vi "SelectDailyData.vi"(8 "Shift":string="中", 10 "Begin_date":string, 11 "End_date":string) -> (2 "output array":string[][](array[string]))   [LabVIEW 2012]
uses:
  <vilib>/addons/database/Auxilliary.llb/DB Tools Cursor Type.ctl
  Global1.vi
  <vilib>/addons/database/Connection.llb/DB Tools Open Connec (Path).vi
  <vilib>/addons/database/Connection.llb/Conn Execute.vi
  <vilib>/addons/database/Recordset.llb/Rec Fetch Recordset Data (R).vi
  <vilib>/addons/database/Recordset.llb/Rec Destroy - Connection.vi
  <vilib>/addons/database/_DB Variant To Data/Database Variant To Data.xnode
  <vilib>/addons/database/NI_Database_API.lvlib
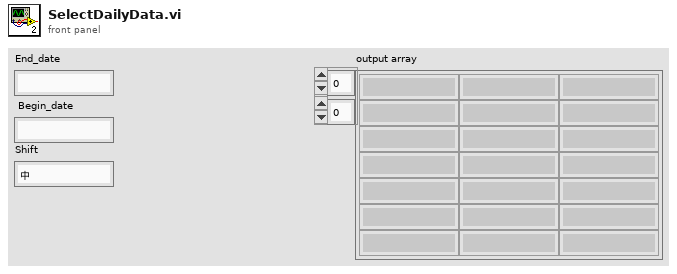
[diagram p1: front panel]
types:
  T1 = typedef "NI_Database_API.lvlib/DB Tools Cursor Type.ctl" = enum16{"forward-only", "keyset", "dynamic", "static"}
  T2 = typedef "NI_Database_API.lvlib/Conn ObjectReference.ctl" = refnum<k1>
  T3 = typedef "NI_Database_API.lvlib/Rec ObjectReference.ctl" = refnum<k1>
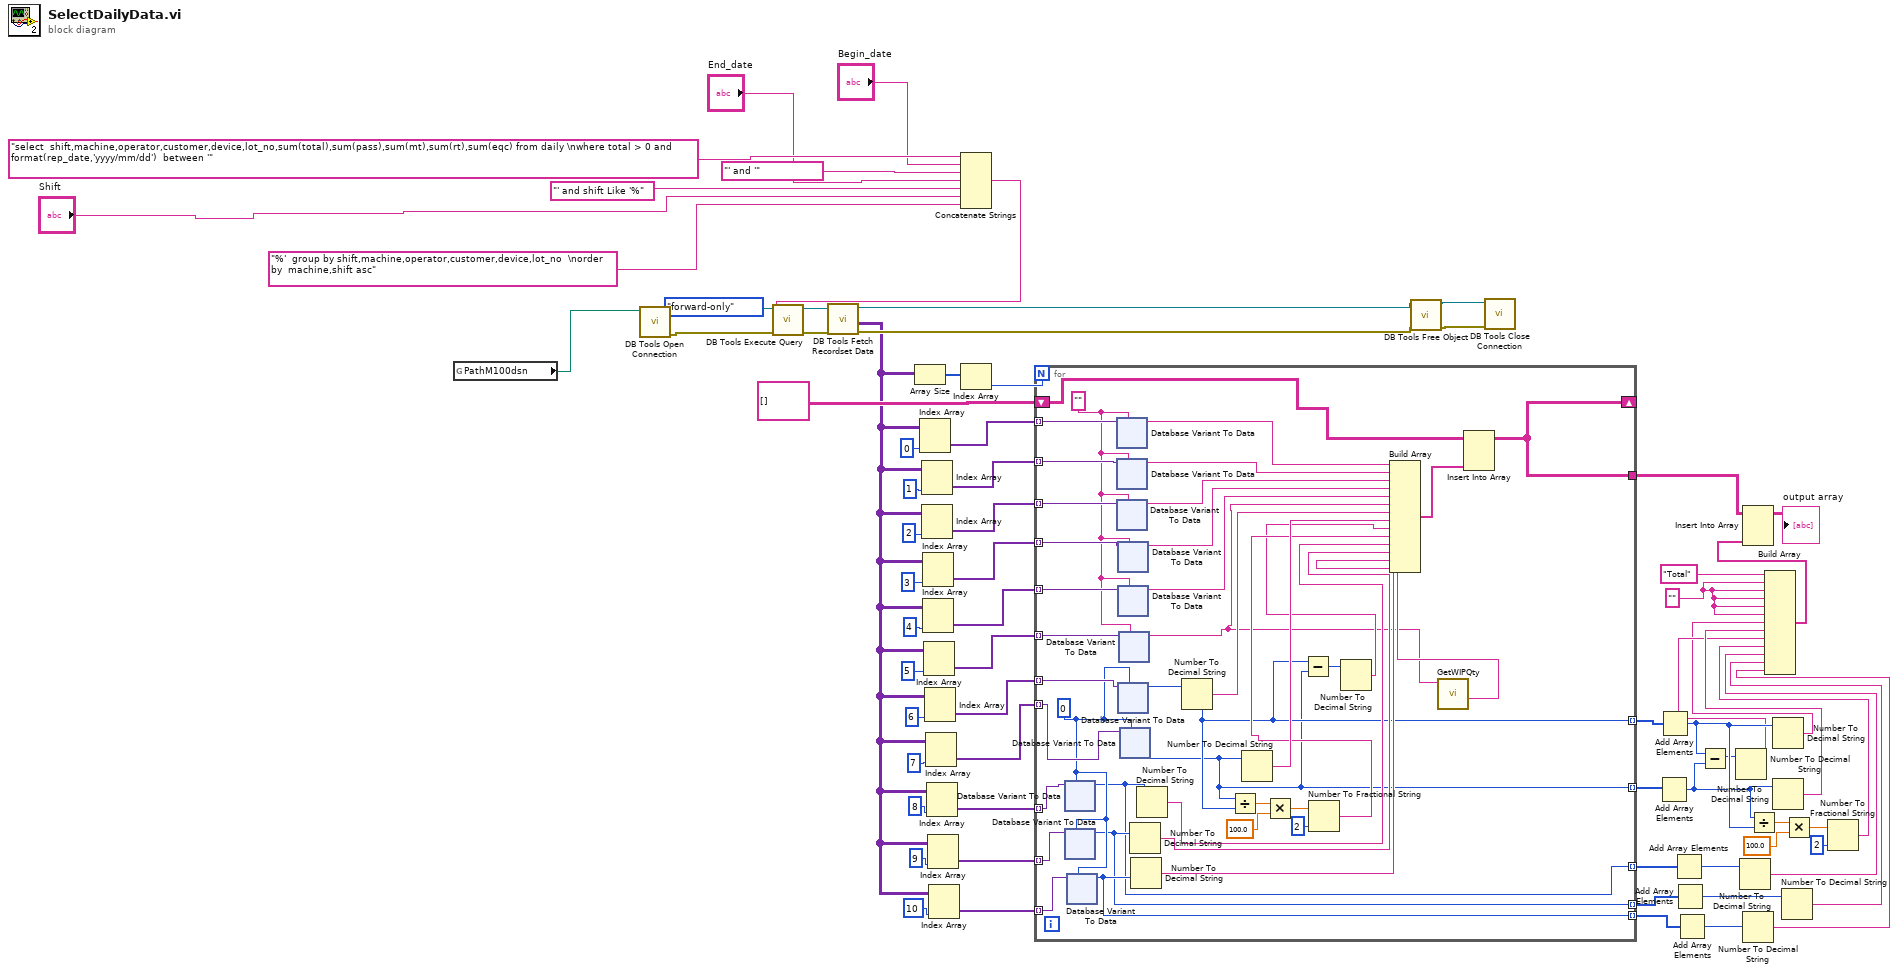
[diagram p0: block diagram]
diagram:
  w47 = "" ("element")
  n1 = global read "Global1.vi" "PathM100dsn"() -> (w1:path)
  n2 = call-poly <vilib>:"DB Tools Open Connection.vi"("connection information"=w1) -> ("error out"=w37:errorcluster, "connection reference"=w38:T2)  [unwired: 7 in]
  n3 = Concatenate Strings("select  shift,machine,operator,customer,device,lot_no,sum(total),sum(pass),sum(mt),sum(rt),sum(eqc) from daily \nwhere total > 0 and  format(rep_date,'yyyy/mm/dd')  between '" ("string"), "Begin_date", "' and '" ("string"), "End_date", "' and shift Like '%" ("string"), "Shift", "%'  group by shift,machine,operator,customer,device,lot_no  \norder by  machine,shift asc" ("string")) -> (w34:string)
  n4 = call-poly <vilib>:"DB Tools Execute Query.vi"("error in (no error)"=w37, "cursor type"=DB_Tools_Cursor_Type."forward-only", "SQL query"=w34, "connection reference"=w38) -> ("error out"=w40:errorcluster, "recordset reference"=w39:T3)  [unwired: 4 in]
  n5 = call-poly <vilib>:"DB Tools Fetch Recordset Data.vi"("error in (no error)"=w40, "recordset reference"=w39) -> ("error out"=w36:errorcluster, "recordset data"=w8:variant[][], "recordset reference out"=w35:T3)  [unwired: 3 in]
  n6 = Array Size(array=w8) -> (size(s)=w71:i32[])
  n7 = Index Array(array=w8, index (col)=0) -> (element=w60:variant[])  [unwired: 1 in]
  n8 = Index Array(array=w8, index (col)=1) -> (element=w67:variant[])  [unwired: 1 in]
  n9 = Index Array(array=w8, index (col)=2) -> (element=w59:variant[])  [unwired: 1 in]
  n10 = Index Array(array=w8, index (col)=3) -> (element=w58:variant[])  [unwired: 1 in]
  n11 = Index Array(array=w8, index (col)=4) -> (element=w57:variant[])  [unwired: 1 in]
  n12 = Index Array(array=w8, index (col)=5) -> (element=w53:variant[])  [unwired: 1 in]
  n13 = Index Array(array=w8, index (col)=6) -> (element=w56:variant[])  [unwired: 1 in]
  n14 = Index Array(array=w8, index (col)=7) -> (element=w55:variant[])  [unwired: 1 in]
  n15 = Index Array(array=w8, index (col)=8) -> (element=w26:variant[])  [unwired: 1 in]
  n16 = Index Array(array=w8, index (col)=9) -> (element=w25:variant[])  [unwired: 1 in]
  n17 = Index Array(array=w8, index (col)=10) -> (element=w24:variant[])  [unwired: 1 in]
  n18 = Index Array(array=w71) -> (element=w70:i32)  [unwired: 1 in]
  n19 = for {
    N: w70 -> [_]
    tunnel: w67 -> [w109] mode=indexing
    tunnel: w55 -> [w111] mode=indexing
    shift-right: [w89] -> _
    shift-left: string[][] [] -> [w95]
    tunnel: w60 -> [w110] mode=indexing
    tunnel: w59 -> [w108] mode=indexing
    tunnel: w58 -> [w107] mode=indexing
    tunnel: w57 -> [w106] mode=indexing
    tunnel: w56 -> [w105] mode=indexing
    tunnel: w53 -> [w102] mode=indexing
    tunnel: [w77] -> w13 mode=indexing
    tunnel: [w76] -> w51 mode=indexing
    tunnel: [w89] -> w32
    tunnel: w26 -> [w88] mode=indexing
    tunnel: w25 -> [w87] mode=indexing
    tunnel: w24 -> [w86] mode=indexing
    tunnel: [w84] -> w21 mode=indexing
    tunnel: [w83] -> w22 mode=indexing
    tunnel: [w82] -> w23 mode=indexing
    w85 = 0
    w101 = ""
    n20 = xnode "Database Variant To Data"("database variant"=w88, "type"=w85) -> ("data"=w82:i32)  [unwired: 1 in, 1 out]
    n21 = xnode "Database Variant To Data"("database variant"=w87, "type"=w85) -> ("data"=w83:i32)  [unwired: 1 in, 1 out]
    n22 = xnode "Database Variant To Data"("database variant"=w86, "type"=w85) -> ("data"=w84:i32)  [unwired: 1 in, 1 out]
    n23 = xnode "Database Variant To Data"("database variant"=w110, "type"=w101) -> ("data"=w94:string)  [unwired: 1 in, 1 out]
    n24 = xnode "Database Variant To Data"("database variant"=w109, "type"=w101) -> ("data"=w93:string)  [unwired: 1 in, 1 out]
    n25 = xnode "Database Variant To Data"("database variant"=w108, "type"=w101) -> ("data"=w90:string)  [unwired: 1 in, 1 out]
    n26 = xnode "Database Variant To Data"("database variant"=w107, "type"=w101) -> ("data"=w92:string)  [unwired: 1 in, 1 out]
    n27 = xnode "Database Variant To Data"("database variant"=w106, "type"=w101) -> ("data"=w91:string)  [unwired: 1 in, 1 out]
    n28 = xnode "Database Variant To Data"("database variant"=w105, "type"=w85) -> ("data"=w77:i32)  [unwired: 1 in, 1 out]
    n29 = xnode "Database Variant To Data"("database variant"=w102, "type"=w101) -> ("data"=w72:string)  [unwired: 1 in, 1 out]
    n30 = xnode "Database Variant To Data"("database variant"=w111, "type"=w85) -> ("data"=w76:i32)  [unwired: 1 in, 1 out]
    n31 = Number To Decimal String(number=w83) -> (decimal integer string=w80:string)  [unwired: 1 in]
    n32 = Number To Decimal String(number=w84) -> (decimal integer string=w81:string)  [unwired: 1 in]
    n33 = Number To Decimal String(number=w82) -> (decimal integer string=w79:string)  [unwired: 1 in]
    n34 = Number To Decimal String(number=w77) -> (decimal integer string=w99:string)  [unwired: 1 in]
    n35 = Divide(x=w76, y=w77) -> (x/y=w103:dbl)
    n36 = Number To Decimal String(number=w76) -> (decimal integer string=w100:string)  [unwired: 1 in]
    n37 = Multiply(x=w103, y=100.0) -> (x*y=w98:dbl)
    n38 = Subtract(x=w77, y=w76) -> (x-y=w75:i32)
    n39 = Number To Fractional String(number=w98, precision (6)=i16 2) -> (F-format string=w78:string)  [unwired: 2 in]
    n40 = Number To Decimal String(number=w75) -> (decimal integer string=w74:string)  [unwired: 1 in]
    n41 = call "GetWIPQty.vi"("Lotno"=w72) -> ("lotno"=w73:string)  [unwired: 6 in, 4 out]
    n42 = Build Array(w94, w93, w90, w92, w91, w72, w99, w100, w74, w78, w79, w80, w81, w73) -> (w96:string[])
    n43 = Insert Into Array(array=w95, new element=w96) -> (w89:string[][])  [unwired: 2 in]
  }
  n44 = call-poly <vilib>:"DB Tools Free Object.vi"("error in (no error)"=w36, "recordset reference"=w35) -> ("error out"=w41:errorcluster, "connection reference"=w42:T2)  [unwired: 8 in]
  n45 = call <vilib>:"DB Tools Close Connection.vi"("error in (no error)"=w41, "connection reference"=w42) -> ()  [unwired: 5 in, 1 out]
  n46 = Add Array Elements(numeric array=w51) -> (sum=w11:i32)
  n47 = Add Array Elements(numeric array=w13) -> (sum=w12:i32)
  n48 = Add Array Elements(numeric array=w23) -> (sum=w20:i32)
  n49 = Add Array Elements(numeric array=w22) -> (sum=w19:i32)
  n50 = Add Array Elements(numeric array=w21) -> (sum=w18:i32)
  n51 = Subtract(x=w12, y=w11) -> (x-y=w10:i32)
  n52 = Number To Decimal String(number=w10) -> (decimal integer string=w9:string)  [unwired: 1 in]
  n53 = Number To Decimal String(number=w20) -> (decimal integer string=w15:string)  [unwired: 1 in]
  n54 = Number To Decimal String(number=w18) -> (decimal integer string=w17:string)  [unwired: 1 in]
  n55 = Divide(x=w11, y=w12) -> (x/y=w45:dbl)
  n56 = Number To Decimal String(number=w12) -> (decimal integer string=w7:string)  [unwired: 1 in]
  n57 = Number To Decimal String(number=w11) -> (decimal integer string=w49:string)  [unwired: 1 in]
  n58 = Number To Decimal String(number=w19) -> (decimal integer string=w16:string)  [unwired: 1 in]
  n59 = Multiply(x=w45, y=100.0) -> (x*y=w44:dbl)
  n60 = Number To Fractional String(number=w44, precision (6)=i16 2) -> (F-format string=w14:string)  [unwired: 2 in]
  n61 = Build Array("Total", w47, w47, w47, w47, w47, w7, w49, w9, w14, w15, w16, w17) -> (w48:string[])
  n62 = Insert Into Array(array=w32, new element=w48) -> (→"output array":string[][])  [unwired: 2 in]
